vi "ICRA2024最后的ratio控制加轨迹跟踪.vi"() -> ()   [LabVIEW 2018]
doc: "Demonstrates the use of the Network Streams functions to send LED status to the myRIO target."
uses:
  <vilib>/Utility/file.llb/Read Delimited Spreadsheet (string).vi
  <vilib>/ErrorRing/Error Ring.xnode
  <vilib>/vision/NI_Vision_Development_Module.lvlib
panel:
  out "期望的ratio":dbl
  out "方向控制量":dbl
  out "速度控制量":dbl
  in  "分裂后的ratio":dbl
  in  "第二个desiredratio":dbl
  in  "第一个desiredratio":dbl
  in  "速度大小":dbl
  in  "终点纵坐标":dbl
  in  "终点横坐标":dbl
  out "实际纵坐标":sgl[](array[numeric])
  out "实际横坐标":sgl[](array[numeric])
  out "实际纵坐标":sgl
  out "实际横坐标":sgl
  out "方向d1":sgl
  out "轨迹跟踪点数":i32
  out "y":dbl
  out "x":dbl
  out "b":dbl[](array[numeric])
  in  "pp":dbl
  out "与目标点的距离":sgl
  in  "guiji":path=path "G:/ICRA-2024-Yuezhen Liu/Labview程序-ICRA2024-YuezhenLiu/small_myRIO_Helmholtz - 1111ke777/zgj轨迹delta为150.txt" caption="call7-8"
  out "Image 8":T1(plugin-control)
  out "ratio误差的绝对值":dbl[](array[numeric])
  in  "pd":dbl
  out "最终的ratio控制量":dbl
  in  "小p":dbl
  out "ratio误差的绝对值":dbl
  out "ratio的误差":dbl[](array[numeric])
  out "第二个前馈":dbl
  out "第一个前馈":dbl
  out "后一个ratio误差":dbl
  out "前一个ratio误差":dbl
  out "第一个i":i32
  out "ratio的误差":dbl
  out "裁剪后的二值图":T1(plugin-control)
  in  "布尔":bool
  in  "ribbon磁场开关":bool=TRUE
  out "面积":sgl[](array[numeric])
  out "面积":sgl
  out "数据总":dbl[][](array[numeric])
  out "i":i32[](array[numeric])
  out "aspect ratio":dbl[](array[numeric])
  out "D2":i32[](array[numeric])
  out "D1":i32[](array[numeric])
  out "field ratio":sgl[](array[numeric])
  out "field ratio":sgl=4.0
  out "时间":i32
  in  "打开数据记录":bool
  out "aspect ratio":dbl
  out "D2":i32
  out "D1":i32
  out "二值图":T1(plugin-control)
  in  "Search Rect (entire image)":T2={"Left"=200, "Top"=120, "Right"=2000, "Bottom"=1920, "Rotation"=0.0} {"Rotation" format="%.2f"; "Left" scale=0.0..1024.0; "Right" scale=0.0..1024.0}
  out "备用的椭圆角度":sgl
  in  "Number of Erosion":i32=10
  out "Image 7":T1(plugin-control)
  in  "Acquisition Control::Acquisition Frame Rate":dbl=19.50304412841797 min=1.4211589097976685 max=44.94382095336914
  out "Stopped":bool
  in  "Stop (F) 2":bool caption="Stop (F)"
  out "Objects 2":T3(array[cluster]) {"Aspect Ratio" format="%.2f"; "Orientation" format="%.2f"; "Area" format="%.2f"; "Object Center"."Y" format="%.2f"; "Object Center"."X" format="%.2f"}
  in  "Settings 2":T4={"Objects"=0, "Threshold"=128, "Reject Border"=FALSE, "Fill Holes"=FALSE, "Min Object Size"=FALSE, "Min Size"=20000, "Max Object Size"=FALSE, "Max Size"=100, "Show Search Area"=FALSE, "Show Center"=TRUE, "Show Bounding Box"=TRUE} {"Objects" items=["Bright Objects", "Dark Objects"]; "Threshold" min=1 max=999999999 step=1; "Max Size" min=1 max=999999999 step=1; "Min Size" min=1 max=999999999 step=1}
  in  "Range 2":cluster{"Lower value":sgl, "Upper value":sgl}={"Lower value"=0.0, "Upper value"=230.0} {"Upper value" format="%.2f"; "Lower value" format="%.2f"}
  in  "Pause":bool
  out "Array":dbl[](array[numeric])
  in  "Parameter Settings":T5(tab)=enum."Ribbon Oscillating Field" caption="Field Types"
  in  "fg":dbl
  in  "pg":dbl
  in  "dg":dbl
  in  "Ag":dbl
  in  "AoOF":dbl
  in  "fo":sgl
  in  "do":sgl
  in  "oo":sgl
  in  "po":sgl
  in  "cc":sgl
  in  "pc":sgl
  in  "wc":sgl
  in  "dc":sgl
  in  "Ac":dbl
  in  "pr":sgl
  in  "Ar":dbl=8.0
  in  "wr":sgl=18.0
  in  "dr":sgl
  in  "Dis phase step":dbl
  in  "Dis phase frequency (Hz)":dbl
  in  "Dis tumbling frequency (Hz)":dbl
  in  "Dis strength(mT)":dbl
  in  "Swa strength (mT)":dbl
  in  "Swa frequency (Hz)":dbl
  in  "Swa pitch angle (deg)":dbl
  in  "Swa direction angle (deg)":dbl
  in  "Swa ratio":dbl=1.0
  in  "Pitch Angle (rotating around Constant, deg)":dbl
  in  "Ratio (A/C)":sgl=4.0
  in  "Direction Angle (deg)":sgl
  in  "Pitch Angle (rotating around Origin, deg)":sgl
  in  "Frequency (Hz)":sgl=10.0
  in  "Strength (mT)":dbl=10.0
  in  "Ar 2":dbl=5.0 caption="Ar"
  in  "ratio":sgl=1.0
  in  "运动方向":sgl
  in  "长轴方向":sgl
  in  "wr  2":sgl=8.0
  in  "速度大小":sgl
  out "Numeric 5":i32
  in  "Stop":bool
  out "error out":errorcluster
  in  "Target IP Address":string="172.22.11.2"
  # "Overview: Magnetic field calculation, and send parameters to myRIO\nInstructions:\n1. Verify the value of Target IP Address. Set Visa resource name.\n2. Ensure RT Main.vi is already running. \n3. Run this VI. Set parameters of magnetic field."
  # "Strength (mT)"
  # "Pitch Angle (deg)"
  # "Direction Angle (deg)"
  # "Frequency (Hz)"
  # "Strength (mT)"
  # "Oscilation Frequency (Hz)"
  # "Oscilation Angle (deg)"
  # "Pitch Angle (deg)"
  # "Direction Angle (deg)"
  # "Strength (mT)"
  # "Frequency (Hz)"
  # "Pitch Angle (deg)"
  # "Direction Angle (deg)"
  # "Conical Angle (deg)"
  # "Strength (mT)"
  # "Frequency (Hz)"
  # "Pitch Angle (deg)"
  # "Direction Angle (deg)"
  # "Strength (mT)"
  # "Tumbling Frequency (Hz)"
  # "Phase Frequency (Hz)"
  # "Phase Step"
  # "Strength (mT)"
  # "Frequency (Hz)"
  # "Pitch Angle (deg)"
  # "Direction Angle (deg)"
  # "Ratio"
  # "Strength (mT)"
  # "Frequency (Hz)"
  # "Ratio (A/C)"
  # "Direction Angle (deg)"
  # "Pitch Angle (rotating around Origin, deg)"
  # "Pitch Angle (rotating around Constant, deg)"
  # "Strength (mT)"
  # "Frequency (Hz)"
  # "Pitch Angle  (deg)"
  # "longaxis"
  # "Direction Angle (deg)"
  # "ratio (l/s)"
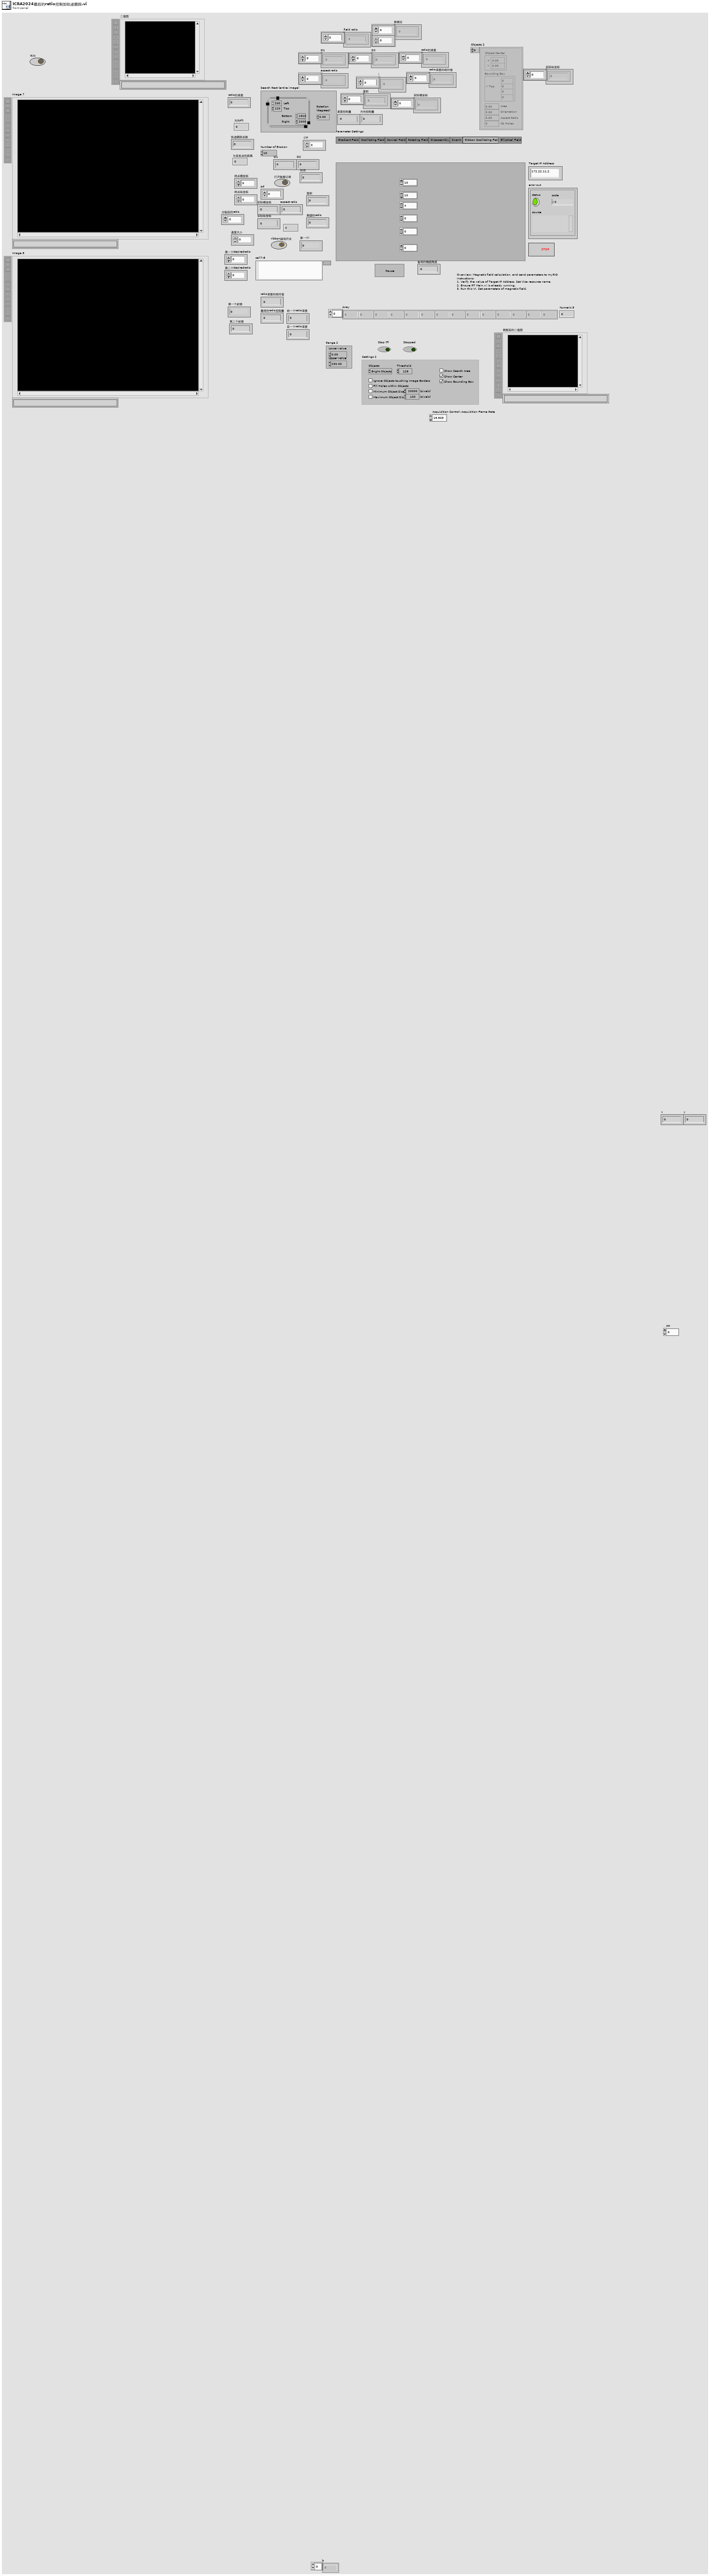
[diagram p1: front panel]
types:
  T1 = typedef "IMAQ Image.ctl" = refnum<image>
  T2 = typedef "IMAQ Rectangle" = cluster{"Left":i32, "Top":i32, "Right":i32, "Bottom":i32, "Rotation":dbl}
  T3 = cluster{"Object Center":cluster{"X":sgl, "Y":sgl}, "Bounding Box":cluster{"X Left":i32, "Y Top":i32, "X Right":i32, "Y Bottom":i32}, "Area":sgl, "Orientation":sgl, "Aspect Ratio":sgl, "Nb Holes":i32}[]
  T4 = cluster{"Objects":u16, "Threshold":i32, "Reject Border":bool, "Fill Holes":bool, "Min Object Size":bool, "Min Size":i32, "Max Object Size":bool, "Max Size":i32, "Show Search Area":bool, "Show Center":bool, "Show Bounding Box":bool}
  T5 = enum32{"Gradient Field ", "Oscillating Field", "Conical Field", "Rotating Field", "Disassembly", "Swarm", "Ribbon Oscillating Field", "Elliptical Field"}
  T6 = cluster{"Left":i32, "Top":i32, "Right":i32, "Bottom":i32}
  T7 = typedef "Image Type" = u32
  T8 = cluster{"Objects[0]":cluster{"Object Center":cluster{"X":sgl, "Y":sgl}, "Bounding Box":cluster{"X Left":i32, "Y Top":i32, "X Right":i32, "Y Bottom":i32}, "Area":sgl, "Orientation":sgl, "Aspect Ratio":sgl, "Nb Holes":i32}, "Objects[1]":cluster{"Object Center":cluster{"X":sgl, "Y":sgl}, "Bounding Box":cluster{"X Left":i32, "Y Top":i32, "X Right":i32, "Y Bottom":i32}, "Area":sgl, "Orientation":sgl, "Aspect Ratio":sgl, "Nb Holes":i32}, "Objects[2]":cluster{"Object Center":cluster{"X":sgl, "Y":sgl}, "Bounding Box":cluster{"X Left":i32, "Y Top":i32, "X Right":i32, "Y Bottom":i32}, "Area":sgl, "Orientation":sgl, "Aspect Ratio":sgl, "Nb Holes":i32}, "Objects[3]":cluster{"Object Center":cluster{"X":sgl, "Y":sgl}, "Bounding Box":cluster{"X Left":i32, "Y Top":i32, "X Right":i32, "Y Bottom":i32}, "Area":sgl, "Orientation":sgl, "Aspect Ratio":sgl, "Nb Holes":i32}, "Objects[4]":cluster{"Object Center":cluster{"X":sgl, "Y":sgl}, "Bounding Box":cluster{"X Left":i32, "Y Top":i32, "X Right":i32, "Y Bottom":i32}, "Area":sgl, "Orientation":sgl, "Aspect Ratio":sgl, "Nb Holes":i32}, "Objects[5]":cluster{"Object Center":cluster{"X":sgl, "Y":sgl}, "Bounding Box":cluster{"X Left":i32, "Y Top":i32, "X Right":i32, "Y Bottom":i32}, "Area":sgl, "Orientation":sgl, "Aspect Ratio":sgl, "Nb Holes":i32}, "Objects[6]":cluster{"Object Center":cluster{"X":sgl, "Y":sgl}, "Bounding Box":cluster{"X Left":i32, "Y Top":i32, "X Right":i32, "Y Bottom":i32}, "Area":sgl, "Orientation":sgl, "Aspect Ratio":sgl, "Nb Holes":i32}, "Objects[7]":cluster{"Object Center":cluster{"X":sgl, "Y":sgl}, "Bounding Box":cluster{"X Left":i32, "Y Top":i32, "X Right":i32, "Y Bottom":i32}, "Area":sgl, "Orientation":sgl, "Aspect Ratio":sgl, "Nb Holes":i32}, "Objects[8]":cluster{"Object Center":cluster{"X":sgl, "Y":sgl}, "Bounding Box":cluster{"X Left":i32, "Y Top":i32, "X Right":i32, "Y Bottom":i32}, "Area":sgl, "Orientation":sgl, "Aspect Ratio":sgl, "Nb Holes":i32}}
  T9 = cluster{"Object Center":cluster{"X":sgl, "Y":sgl}, "Bounding Box":cluster{"X Left":i32, "Y Top":i32, "X Right":i32, "Y Bottom":i32}, "Area":sgl, "Orientation":sgl, "Aspect Ratio":sgl, "Nb Holes":i32}
  T10 = cluster{"X Left":i32, "Y Top":i32, "X Right":i32, "Y Bottom":i32}
  T11 = typedef "ROI Descriptor" = cluster{"Global Rectangle":i32[], "Contours":cluster{"ID":enum32{"External", "Internal"}, "Type":u32, "Coordinates":i32[]}[]}
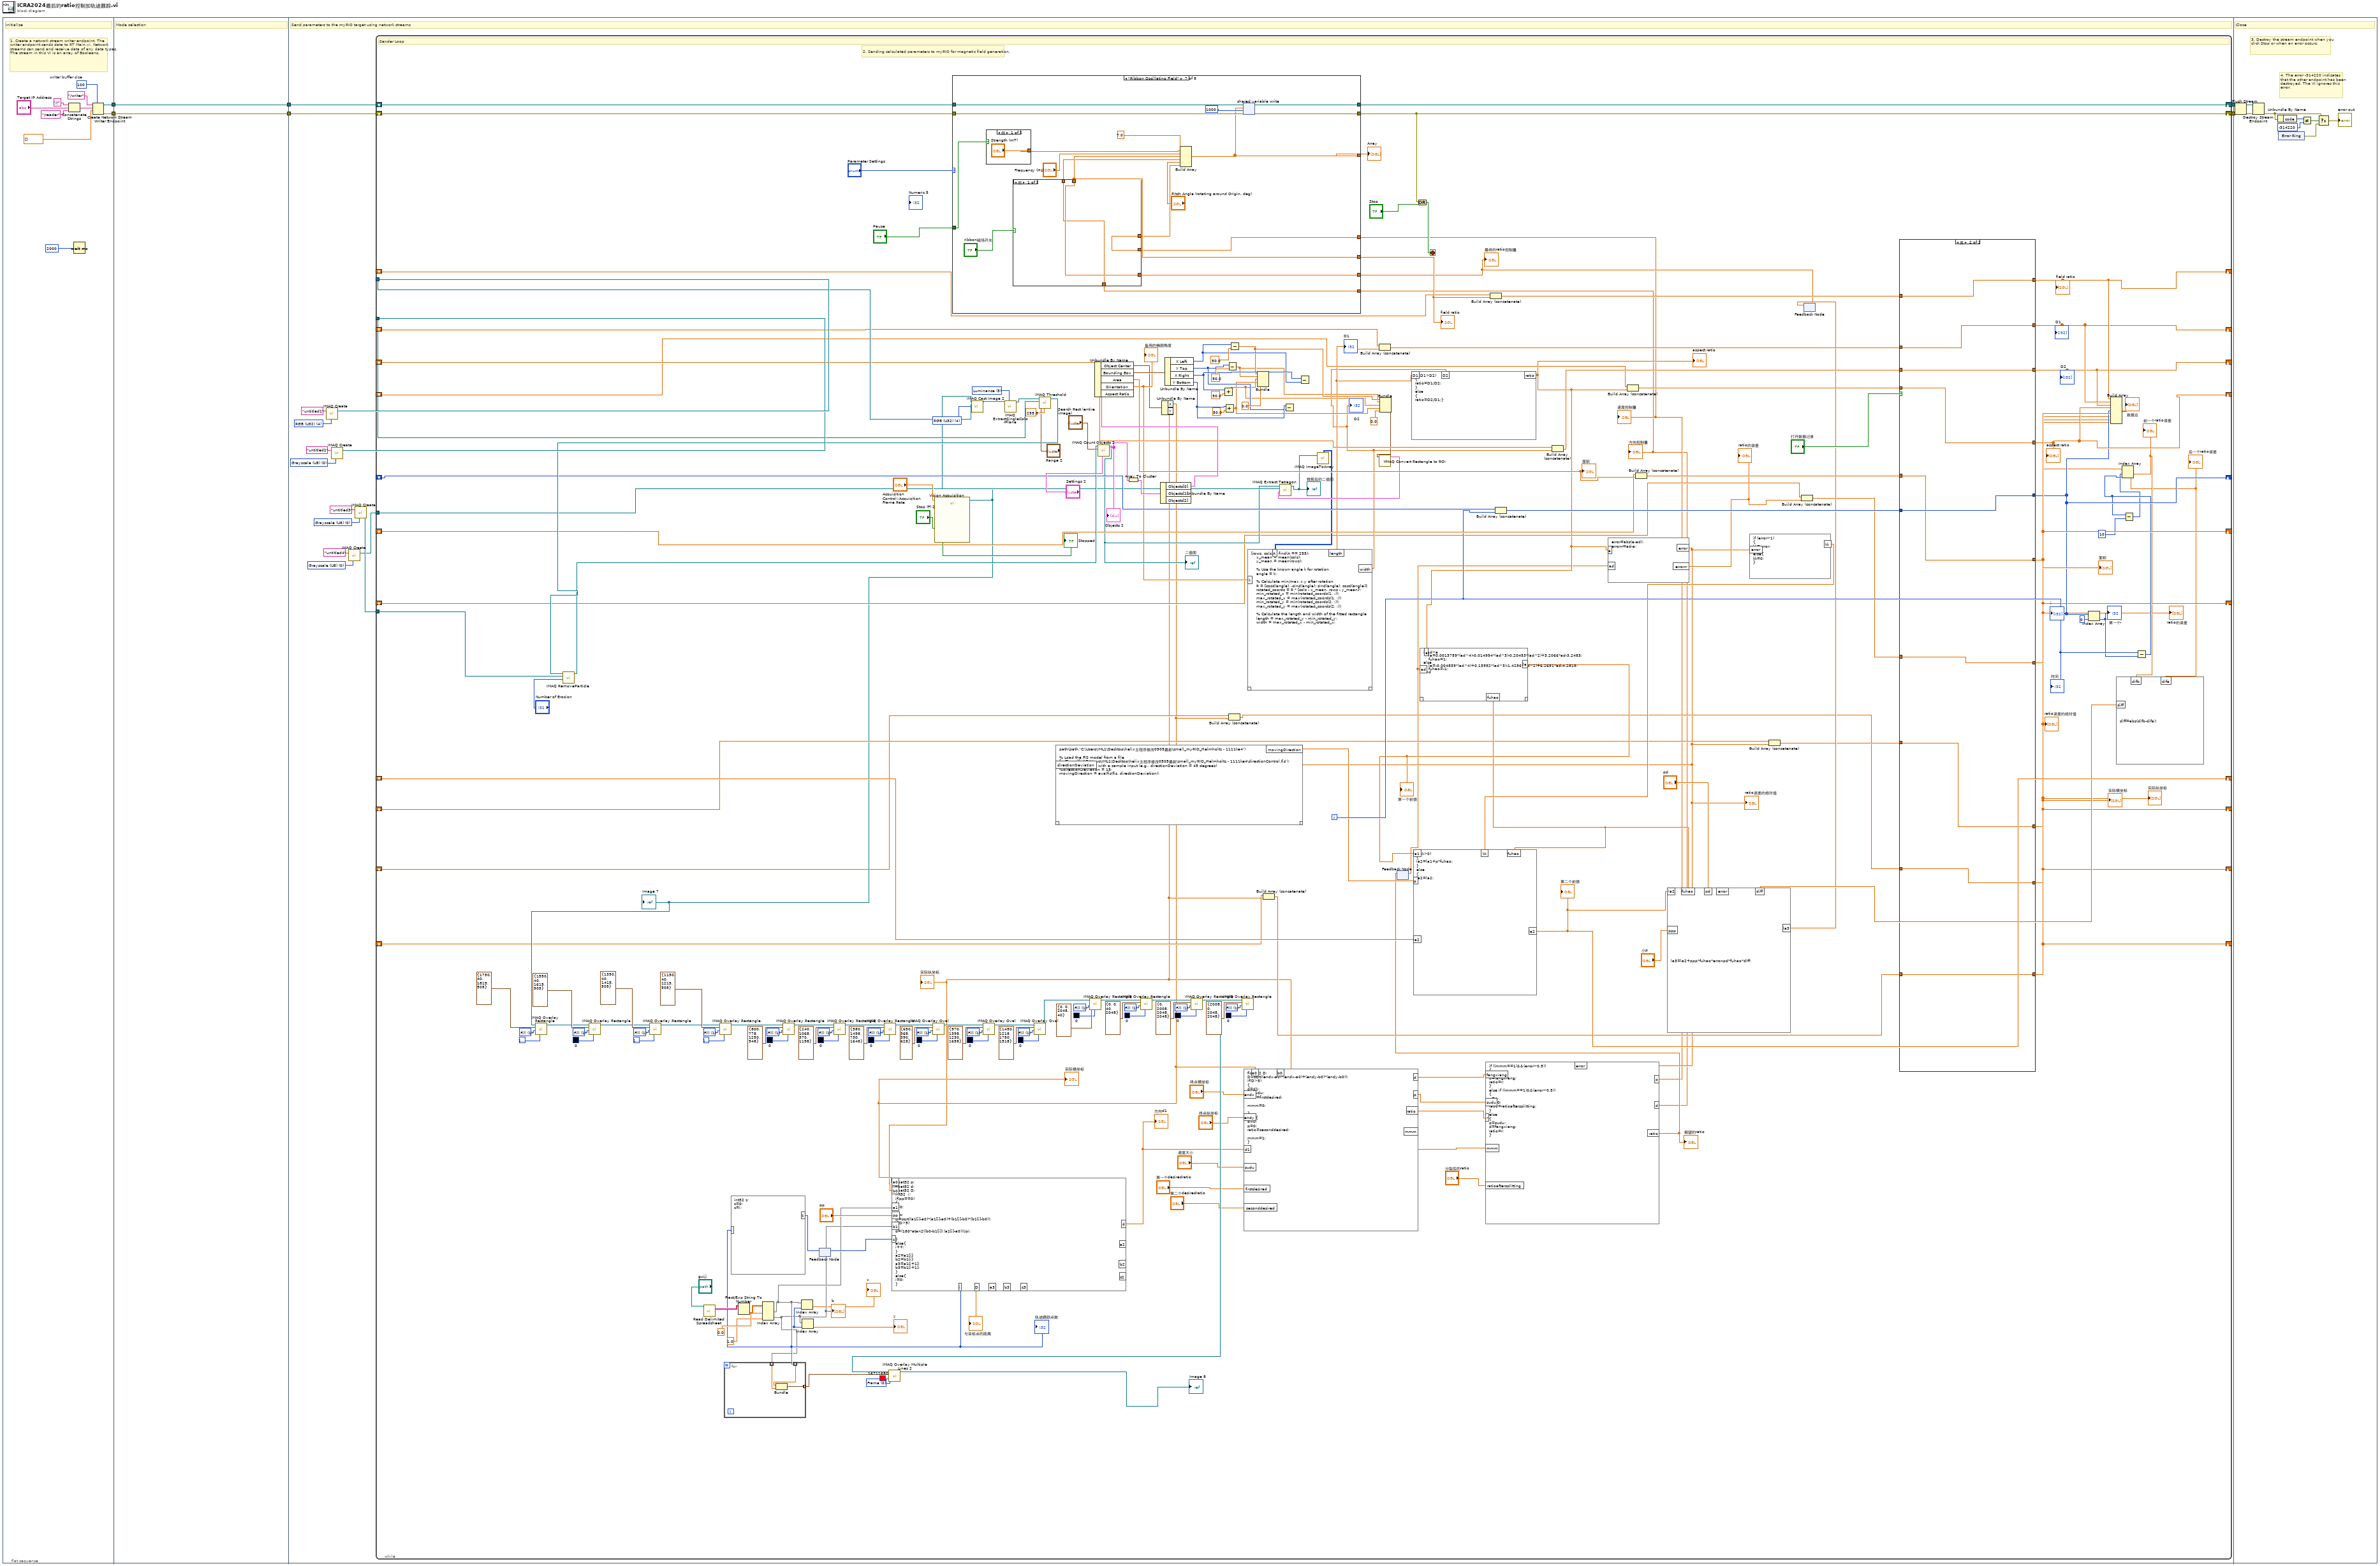
[diagram p0: block diagram]
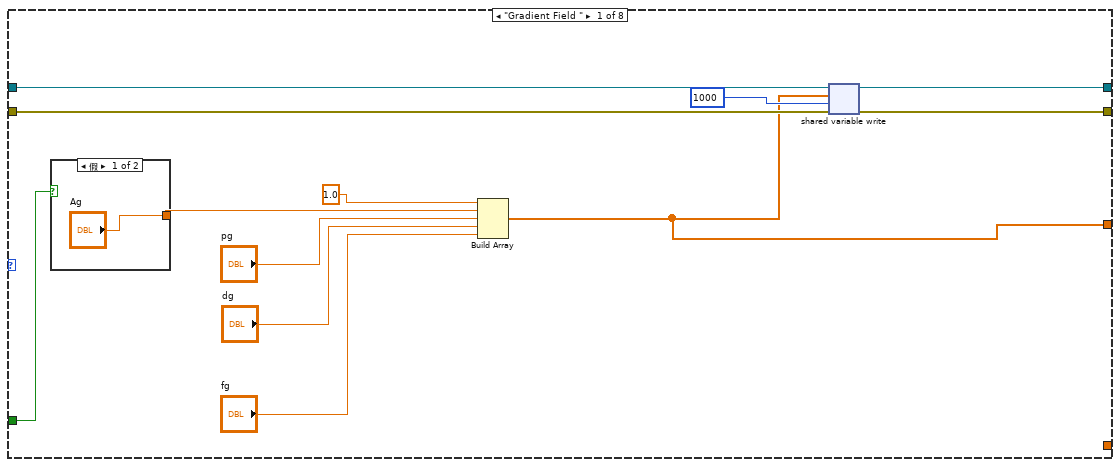
[diagram p3: hidden frame]
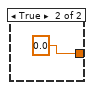
[diagram p4: hidden frame]
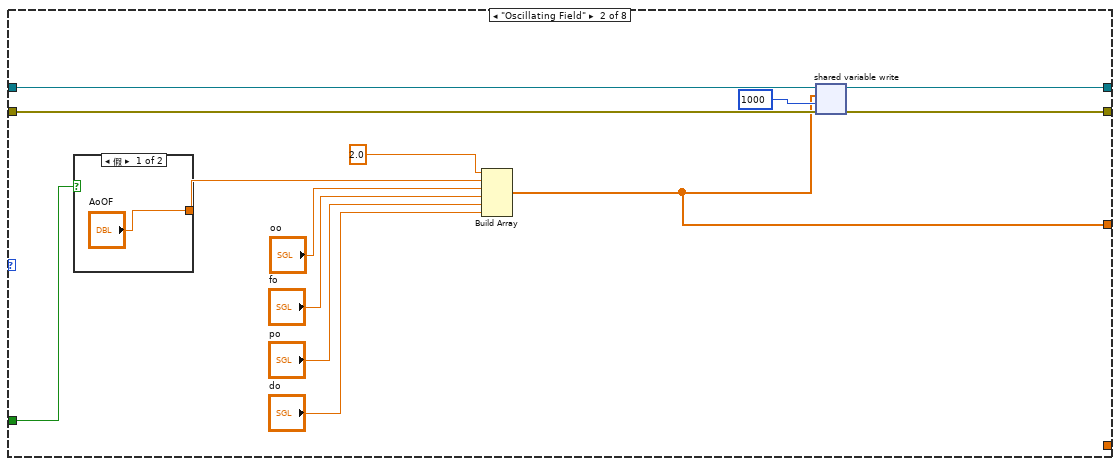
[diagram p5: hidden frame]
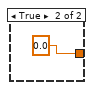
[diagram p6: hidden frame]
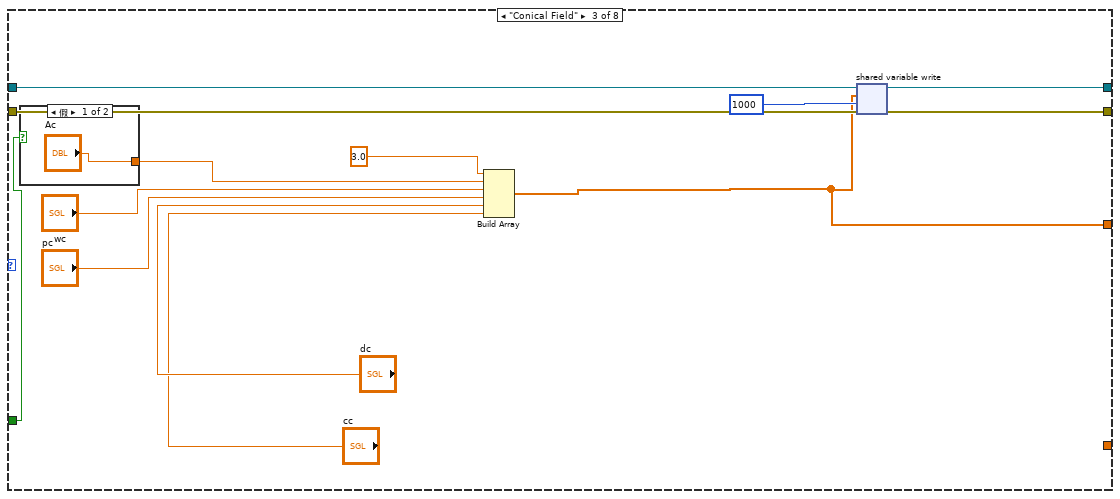
[diagram p7: hidden frame]
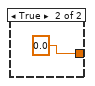
[diagram p8: hidden frame]
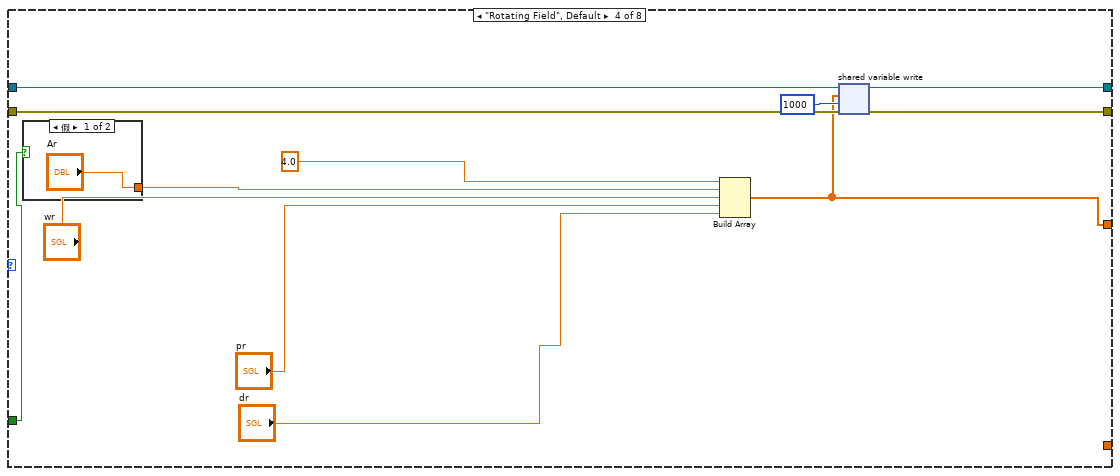
[diagram p9: hidden frame]
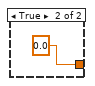
[diagram p10: hidden frame]
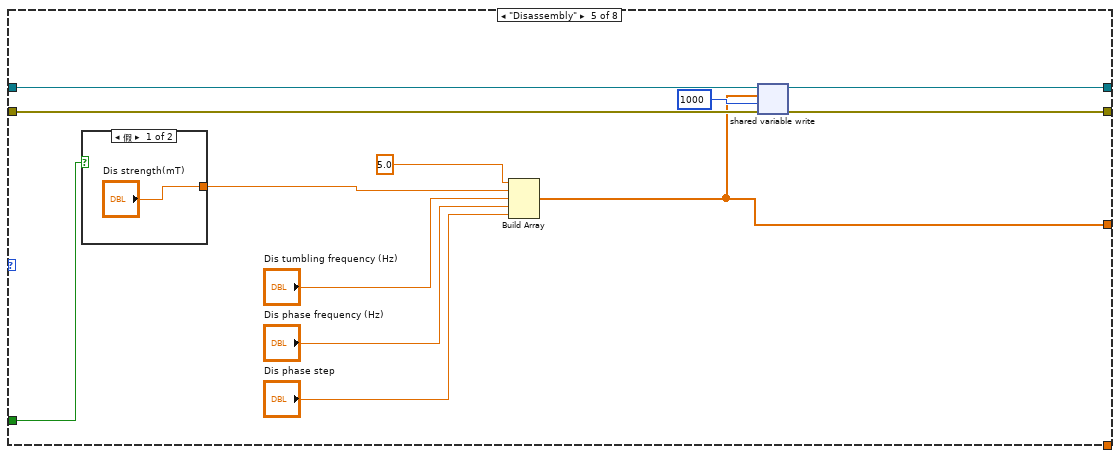
[diagram p11: hidden frame]
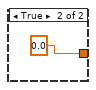
[diagram p12: hidden frame]
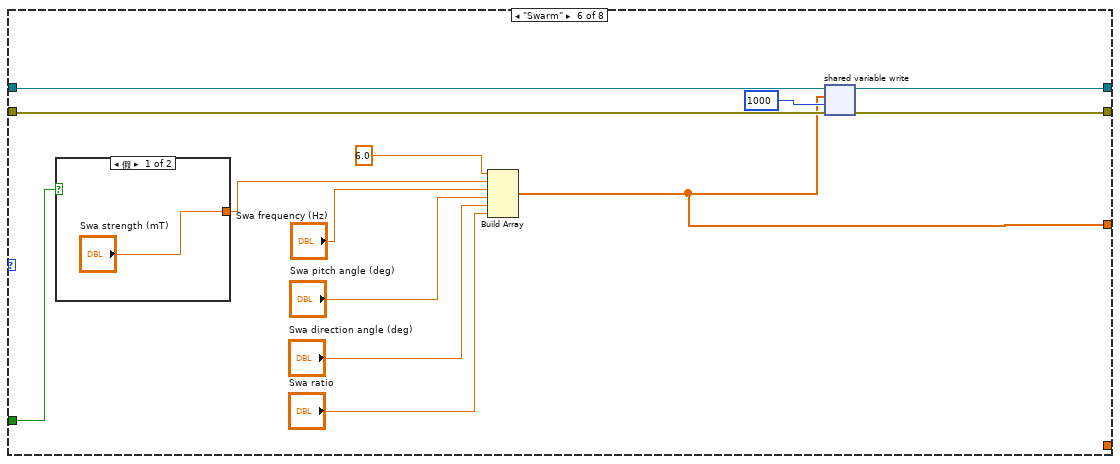
[diagram p13: hidden frame]
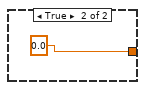
[diagram p14: hidden frame]
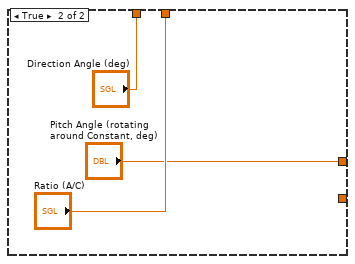
[diagram p15: hidden frame]
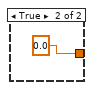
[diagram p16: hidden frame]
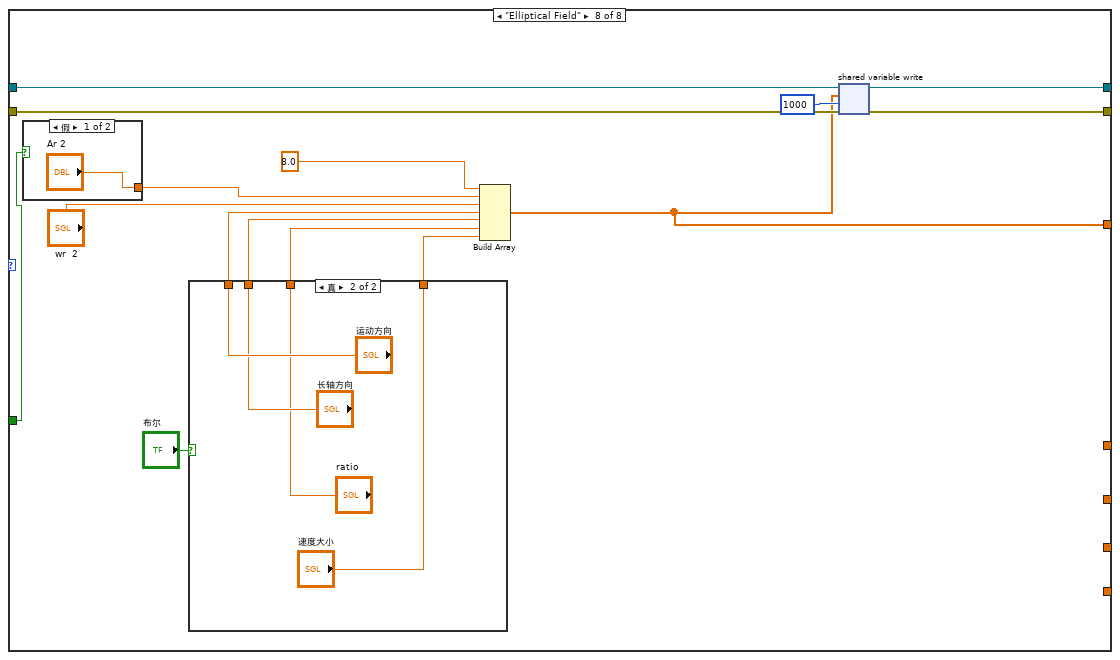
[diagram p17: hidden frame]
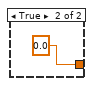
[diagram p19: hidden frame]
diagram:
  n1 = flat-sequence {
    tunnel: [w11] -> w2
    tunnel: [w10] -> w1
    tunnel: [w18] -> w4
    tunnel: [w17] -> w3
    tunnel: w1 -> [w17]
    tunnel: w2 -> [w18]
    tunnel: [w32] -> w6
    tunnel: w4 -> [w34]
    tunnel: [w31] -> w5
    tunnel: w3 -> [w33]
    tunnel: w6 -> [w393]
    tunnel: w5 -> [w390]
    frame #0 {
      w9 = 100  # writer buffer size
      # "1. Create a network stream writer endpoint. The writer endpoint sends data to RT Main.vi. Network streams can send and receive data of any data types. The stream in this VI is an array of Booleans."
      # "Initialize"
      n2 = Concatenate Strings("//", "Target IP Address", "/reader") -> (w16:string)
      n3 = Wait (ms)(milliseconds to wait=2000) -> ()  [unwired: 1 out]
      n4 = Create Network Stream Writer Endpoint(7:w9, 9:dbl[] [], 10:w16, 11:"/writer" ("reader name")) -> (0:w10:errorcluster, 3:w11:refnum<k21>)  [unwired: 3 in]
    }
    frame #1 {
      # "Mode selection"
    }
    frame #2 {
      w20 = T7 0 items=["Grayscale (U8)", "Grayscale (I16)", "Grayscale (SGL)", "Complex (CSG)", "RGB (U32)", "HSL (U32)", "RGB (U64)", "Grayscale (U16)"] ("Image Type")
      w23 = T7 0 items=["Grayscale (U8)", "Grayscale (I16)", "Grayscale (SGL)", "Complex (CSG)", "RGB (U32)", "HSL (U32)", "RGB (U64)", "Grayscale (U16)"] ("Image Type")
      w27 = T7 0 items=["Grayscale (U8)", "Grayscale (I16)", "Grayscale (SGL)", "Complex (CSG)", "RGB (U32)", "HSL (U32)", "RGB (U64)", "Grayscale (U16)"] ("Image Type")
      w29 = T7 4 items=["Grayscale (U8)", "Grayscale (I16)", "Grayscale (SGL)", "Complex (CSG)", "RGB (U32)", "HSL (U32)", "RGB (U64)", "Grayscale (U16)"] ("Image Type")
      # "Send parameters to the myRIO target using network streams"
      n5 = call "IMAQ Create"("Image Name"="untitled1", "Image Type"=w29) -> ("New Image"=w26:T1)  [unwired: 3 in, 1 out]
      n6 = call "IMAQ Create"("Image Name"="untitled2", "Image Type"=w27) -> ("New Image"=w25:T1)  [unwired: 3 in, 1 out]
      n7 = call "IMAQ Create"("Image Name"="untitled4", "Image Type"=w20) -> ("New Image"=w19:T1)  [unwired: 3 in, 1 out]
      n8 = call "IMAQ Create"("Image Name"="untitled3", "Image Type"=w23) -> ("New Image"=w22:T1)  [unwired: 3 in, 1 out]
      n9 = while {
        shift-right: [w232] -> w31
        shift-left: w33 -> [w234]
        shift-right: [w233] -> w32
        shift-left: w34 -> [w235]
        tunnel: w25 -> [w223]
        tunnel: w26 -> [w218]
        tunnel: w22 -> [w207]
        shift-right: [w185] -> _
        shift-left: _ -> [w194]
        shift-right: [w184] -> _
        shift-left: _ -> [w192]
        shift-right: [w183] -> _
        shift-left: _ -> [w190]
        shift-right: [w164] -> _
        shift-left: _ -> [w188]
        shift-right: [w163] -> _
        shift-left: _ -> [w186]
        shift-right: [w179] -> _
        shift-left: _ -> [w178]
        tunnel: w19 -> [w177]
        shift-right: [w153] -> _
        shift-left: _ -> [w154]
        shift-right: [w151] -> _
        shift-left: _ -> [w150]
        shift-right: [w135] -> _
        shift-left: _ -> [w136]
        shift-right: [w54] -> _
        shift-left: _ -> [w57]
        shift-right: [w53] -> _
        shift-left: _ -> [w55]
        i -> [w161]
        stop <- w222 stop-if-true
        w62 = u32 0 items=["Frame", "Fill"] ("Drawing Mode (Frame)")
        w81 = u32 1 items=["Frame", "Fill", "Highlight"] ("Drawing Mode (Frame)")
        w84 = u32 1 items=["Frame", "Fill", "Highlight"] ("Drawing Mode (Frame)")
        w87 = u32 1 items=["Frame", "Fill", "Highlight"] ("Drawing Mode (Frame)")
        w90 = u32 1 items=["Frame", "Fill", "Highlight"] ("Drawing Mode (Frame)")
        w97 = u32 1 items=["Frame", "Fill"] ("Drawing Mode (Frame)")
        w100 = u32 1 items=["Frame", "Fill"] ("Drawing Mode (Frame)")
        w105 = u32 1 items=["Frame", "Fill"] ("Drawing Mode (Frame)")
        w117 = u32 1 items=["Frame", "Fill", "Highlight"] ("Drawing Mode (Frame)")
        w110 = u32 1 items=["Frame", "Fill"] ("Drawing Mode (Frame)")
        w120 = u32 1 items=["Frame", "Fill", "Highlight"] ("Drawing Mode (Frame)")
        w125 = u32 1 items=["Frame", "Fill", "Highlight"] ("Drawing Mode (Frame)")
        w128 = u32 1 items=["Frame", "Fill", "Highlight"] ("Drawing Mode (Frame)")
        w131 = u32 1 items=["Frame", "Fill", "Highlight"] ("Drawing Mode (Frame)")
        w134 = u32 1 items=["Frame", "Fill", "Highlight"] ("Drawing Mode (Frame)")
        w217 = T7 4 items=["Grayscale (U8)", "Grayscale (I16)", "Grayscale (SGL)", "Complex (CSG)", "RGB (U32)", "HSL (U32)", "RGB (U64)", "Grayscale (U16)"] ("Image Type")
        w228 = 5 items=["Red", "Green", "Blue", "Hue", "Saturation", "Luminance", "Value", "Intensity"] ("Color Plane")
        # "2. Sending calculated parameters to myRIO for magnetic field generation."
        # "Sender Loop"
        n10 = call-poly <vilib>:"Read Delimited Spreadsheet.vi"("file path (dialog if empty)"="guiji") -> ("all rows"=w77:string[][])  [unwired: 9 in, 5 out]
        n11 = Fract/Exp String To Number(string=w77) -> (number=w76:dbl[][])  [unwired: 3 in, 1 out]
        n12 = Index Array(array=w76, index (col) #1=0.0, index (col) #2=1.0) -> (element #1=w69:dbl[], element #2=w67:dbl[])  [unwired: 2 in]
        "b" <- w67
        n13 = for {
          tunnel: w69 -> [w239] mode=indexing
          tunnel: w67 -> [w238] mode=indexing
          tunnel: [w237] -> w64 mode=indexing
          n14 = Bundle("String"=w239, "String"=w238) -> (w237:cluster{"String":dbl, "String":dbl})  [unwired: 1 in]
        }
        n15 = feedback #1() -> (w72:i32)  [unwired: 1 in]
        n16 = call "Vision Acquisition"("Acquisition Control::Acquisition Frame Rate"="Acquisition Control::Acquisition Frame Rate", "Stop (F)"="Stop (F) 2") -> ("Image Out"=w79:T1, "Stopped"=→"Stopped":bool)  [unwired: 23 in, 1 out]
        "Image 7" <- w79
        n17 = call "IMAQ Overlay Rectangle"("Color"=u32 16777222, "Drawing Mode (Frame)"=w128, "Rectangle"=T6 {"Left"=1750, "Top"=40, "Right"=1815, "Bottom"=505}, "Image"=w79) -> ("Image Out"=w108:T1)  [unwired: 6 in, 1 out]
        n18 = call "IMAQ Overlay Rectangle"("Color"=u32 0, "Drawing Mode (Frame)"=w125, "Rectangle"=T6 {"Left"=1550, "Top"=40, "Right"=1615, "Bottom"=505}, "Image"=w108) -> ("Image Out"=w122:T1)  [unwired: 6 in, 1 out]
        n19 = call "IMAQ Overlay Rectangle"("Color"=u32 16777222, "Drawing Mode (Frame)"=w131, "Rectangle"=T6 {"Left"=1350, "Top"=40, "Right"=1415, "Bottom"=505}, "Image"=w122) -> ("Image Out"=w121:T1)  [unwired: 6 in, 1 out]
        n20 = call "IMAQ Overlay Rectangle"("Color"=u32 16777222, "Drawing Mode (Frame)"=w134, "Rectangle"=T6 {"Left"=1150, "Top"=40, "Right"=1215, "Bottom"=505}, "Image"=w121) -> ("Image Out"=w109:T1)  [unwired: 6 in, 1 out]
        n21 = call "IMAQ Overlay Rectangle"("Color"=u32 0, "Drawing Mode (Frame)"=w120, "Rectangle"=T6 {"Left"=800, "Top"=778, "Right"=1250, "Bottom"=948}, "Image"=w109) -> ("Image Out"=w113:T1)  [unwired: 6 in, 1 out]
        n22 = call "IMAQ Overlay Rectangle"("Color"=u32 0, "Drawing Mode (Frame)"=w110, "Rectangle"=T6 {"Left"=240, "Top"=1068, "Right"=370, "Bottom"=1198}, "Image"=w113) -> ("Image Out"=w114:T1)  [unwired: 6 in, 1 out]
        n23 = call "IMAQ Overlay Rectangle"("Color"=u32 0, "Drawing Mode (Frame)"=w117, "Rectangle"=T6 {"Left"=580, "Top"=1498, "Right"=730, "Bottom"=1648}, "Image"=w114) -> ("Image Out"=w107:T1)  [unwired: 6 in, 1 out]
        n24 = call "IMAQ Overlay Oval"("Color"=u32 0, "Drawing Mode (Frame)"=w105, "Bounding Rectangle"=T6 {"Left"=650, "Top"=368, "Right"=390, "Bottom"=628}, "Image"=w107) -> ("Image Out"=w102:T1)  [unwired: 6 in, 1 out]
        n25 = call "IMAQ Cast Image 2"("Image Src"=w79, "Image Dst"=w218, "Image Type"=w217) -> ("Image Dst Out"=w219:T1)  [unwired: 11 in, 1 out]
        n26 = call "IMAQ Overlay Oval"("Color"=u32 0, "Drawing Mode (Frame)"=w100, "Bounding Rectangle"=T6 {"Left"=970, "Top"=1398, "Right"=1230, "Bottom"=1658}, "Image"=w102) -> ("Image Out"=w103:T1)  [unwired: 6 in, 1 out]
        n27 = call "IMAQ ExtractSingleColorPlane"("Color Plane"=w228, "Image Src"=w219) -> ("Image Dst Out"=w205:T1)  [unwired: 8 in, 1 out]
        n28 = call "IMAQ Overlay Oval"("Color"=u32 0, "Drawing Mode (Frame)"=w97, "Bounding Rectangle"=T6 {"Left"=1450, "Top"=1218, "Right"=1750, "Bottom"=1518}, "Image"=w103) -> ("Image Out"=w95:T1)  [unwired: 6 in, 1 out]
        n29 = call "IMAQ Threshold"("Replace Value"=sgl 255.0, "Range"="Range 2", "Image Dst"=w223, "Image Src"=w205) -> ("Image Dst Out"=w208:T1)  [unwired: 6 in, 1 out]
        n30 = call "IMAQ RemoveParticle"("Number of Erosion"="Number of Erosion", "Image Dst"=w207, "Image Src"=w208) -> ("Image Dst Out"=w200:T1)  [unwired: 7 in, 1 out]
        n31 = call "IMAQ Overlay Rectangle"("Color"=u32 0, "Drawing Mode (Frame)"=w90, "Rectangle"=T6 {"Left"=0, "Top"=0, "Right"=2048, "Bottom"=40}, "Image"=w95) -> ("Image Out"=w94:T1)  [unwired: 6 in, 1 out]
        n32 = call "IMAQ Count Objects 2"("Settings"="Settings 2", "Search Rect (entire image)"="Search Rect (entire image)", "Image"=w200) -> ("Image Out"=w176:T1, "Objects"=w224:T3)  [unwired: 4 in, 3 out]
        "Objects 2" <- w224
        "二值图" <- w176
        n33 = Array To Cluster(array=w224) -> (cluster=w210:T8)
        n34 = call "IMAQ Overlay Rectangle"("Color"=u32 0, "Drawing Mode (Frame)"=w87, "Rectangle"=T6 {"Left"=0, "Top"=0, "Right"=40, "Bottom"=2048}, "Image"=w94) -> ("Image Out"=w93:T1)  [unwired: 6 in, 1 out]
        n35 = Unbundle By Name(w210) -> ("Objects[0]"=w209:T9)  [unwired: 2 out]
        n36 = Unbundle By Name(w209) -> ("Object Center"=w59:cluster{"X":sgl, "Y":sgl}, "Bounding Box"=w216:T10, "Area"=w181:sgl, "Orientation"=w159:sgl)  [unwired: 1 out]
        "备用的椭圆角度" <- w159
        "面积" <- w181
        n37 = Unbundle By Name(w59) -> ("X"=w48:sgl, "Y"=w47:sgl)
        "实际横坐标" <- w48
        "实际纵坐标" <- w47
        n38 = formula code="float32 p;\nfloat32 d;\nfloat32 D;\nint32  i;\nif(pp==0)\n{\ni=0;\n\ni=z;\nD=sqrt((a1[i]-a0)*(a1[i]-a0)+(b1[i]-b0)*(b1[i]-b0));\nif(D>5)\n{\nd=(180*atan2((b0-b1[i]),(a1[i]-a0)))/pi;\n\n}\nelse{\ni++;\n}\na2=a1[i];\nb2=b1[i];\na3=a1[i+1];\nb3=b1[i+1];\n}\nelse{\ni=0;\n}"("a0"=w48, "b0"=w47, "a1"=w69, "b1"=w67, "z"=w72, "pp"="pp") -> ("i"=w68:i32, "D"=→"与目标点的距离":sgl, "d"=w50:sgl)  [unwired: 6 out]
        "轨迹跟踪点数" <- w68
        "方向d1" <- w50
        n39 = formula code="int32 z;\nz=0;\nz=i;"("i"=w68) -> ("z"=w73:i32)
        n40 = Index Array(array=w69, index=w68) -> (element=→"x":dbl)
        n41 = Index Array(array=w67, index=w68) -> (element=→"y":dbl)
        n42 = feedback-in #1(w73) -> ()
        n43 = Unbundle By Name(w216) -> ("X Left"=w202:i32, "Y Top"=w198:i32, "X Right"=w203:i32, "Y Bottom"=w199:i32)
        n44 = call "IMAQ Overlay Rectangle"("Color"=u32 0, "Drawing Mode (Frame)"=w84, "Rectangle"=T6 {"Left"=0, "Top"=2008, "Right"=2048, "Bottom"=2048}, "Image"=w93) -> ("Image Out"=w92:T1)  [unwired: 6 in, 1 out]
        n45 = Add(x=w203, y=50.0) -> (x+y=w171:dbl)
        n46 = Add(x=w199, y=50.0) -> (x+y=w170:dbl)
        n47 = Subtract(x=w198, y=50.0) -> (x-y=w172:dbl)
        n48 = Build Array (concatenate)(w57, w48) -> (w58:sgl[])
        n49 = Subtract(x=w202, y=50.0) -> (x-y=w173:dbl)
        n50 = call "IMAQ Overlay Rectangle"("Color"=u32 0, "Drawing Mode (Frame)"=w81, "Rectangle"=T6 {"Left"=2008, "Top"=0, "Right"=2048, "Bottom"=2048}, "Image"=w92) -> ("Image Out"=w61:T1)  [unwired: 6 in, 1 out]
        n51 = call "IMAQ Overlay Multiple Lines 2"("Image"=w61, "Line End Points"=w64, "Drawing Mode (Frame)"=w62, "Color"=u32 16711680) -> ("Image Out"=→"Image 8":T1)  [unwired: 10 in, 1 out]
        n52 = formula code="float32 D;\nD=sqrt((endx-a0)*(endx-a0)+(endy-b0)*(endy-b0));\nif(D>5)\n{\nd=d1;\np=sudu;\nratio=firstdesired;\n\nmmm=0;\n\n}\nelse{\nd=0;\np=0;\nratio=seconddesired;\n\nmmm=1;\n}"("endx"="终点横坐标", "endy"="终点纵坐标", "d1"=w50, "sudu"="速度大小", "firstdesired"="第一个desiredratio", "seconddesired"="第二个desiredratio", "a0"=w48, "b0"=w47) -> ("p"=w43:dbl, "ratio"=w41:dbl, "d"=w42:dbl, "mmm"=w44:dbl)
        n53 = Bundle(w173, w172, w171, w170, 0.0) -> ()  [unwired: 1 in, 1 out]
        n54 = Build Array (concatenate)(w55, w47) -> (w56:sgl[])
        n55 = Subtract(x=w199, y=w198) -> ()  [unwired: 1 out]
        n56 = Subtract(x=w203, y=w202) -> ()  [unwired: 1 out]
        n57 = Bundle(w173, w172, w171, w170, 0.0) -> (w168:cluster{dbl, dbl, dbl, dbl, dbl})  [unwired: 1 in]
        n58 = call "IMAQ Convert Rectangle to ROI"("Rectangle"=w168) -> ("ROI Descriptor"=w174:T11)  [unwired: 8 in, 1 out]
        n59 = call-poly "IMAQ Extract Tetragon"("ROI Descriptor"=w174, "Image Dst"=w177, "Image Src"=w176) -> ("Image Dst Out"=w175:T1)  [unwired: 7 in, 1 out]
        "裁剪后的二值图" <- w175
        n60 = call "IMAQ ImageToArray"("Image"=w175) -> ("Image Pixels (U8)"=w167:u8[][])  [unwired: 3 in, 4 out]
        n61 = script code="[rows, cols] = find(A == 255);\n    x_mean = mean(cols);\n    y_mean = mean(rows);\n\n    % Use the known angle k for rotation\n    angle = k;\n\n    % Calculate min/max x,y after rotation\n    R = [cosd(angle), -sind(angle); sind(angle), cosd(angle)];\n    rotated_coords = R * [cols - x_mean, rows - y_mean]';\n    min_rotated_x = min(rotated_coords(1, :));\n    max_rotated_x = max(rotated_coords(1, :));\n    min_rotated_y = min(rotated_coords(2, :));\n    max_rotated_y = max(rotated_coords(2, :));\n\n    % Calculate the length and width of the fitted rectangle\n    length = max_rotated_y - min_rotated_y;\n    width = max_rotated_x - min_rotated_x;"("A"=w167, "k"=w159) -> ("length"=w166:dbl, "width"=w165:dbl)  [unwired: 1 in, 1 out]
        "D1" <- w166
        "D2" <- w165
        n62 = Build Array (concatenate)(w192, w166) -> (w193:dbl[])
        n63 = feedback #2() -> (w37:dbl)  [unwired: 1 in]
        n64 = formula code="if (D1>D2)\n{\nratio=D1/D2;\n}\nelse\n{\nratio=D2/D1;}"("D1"=w166, "D2"=w165) -> ("ratio"=w139:dbl)
        "aspect ratio" <- w139
        n65 = script code="if ad>a\n    la=0.0013759*(ad^4)-0.014994*(ad^3)-0.20453*(ad^2)+3.2066*ad-3.2483;\n    fuhao=1;\nelse\n    la=-0.004839*(ad^4)+0.13992*(ad^3)-1.4256*(ad^2)+6.2651*ad-4.2815;\n    fuhao=-1;\nend"("a"=w139, "ad"=w37) -> ("la"=w141:dbl, "fuhao"=w140:dbl)  [unwired: 1 in, 1 out]
        "第一个前馈" <- w141
        n66 = Build Array (concatenate)(w186, w161) -> (w187:i32[])
        n67 = Build Array (concatenate)(w190, w165) -> (w191:dbl[])
        n68 = formula code="error=abs(a-ad);\nerrorrr=ad-a;"("a"=w139, "ad"=w37) -> ("error"=w40:dbl, "errorrr"=w146:dbl)
        "ratio的误差" <- w146
        "ratio误差的绝对值" <- w40
        n69 = script code="path(path,'C:\\Users\\IML1\\Desktop\\helix主程序修改0505最新\\small_myRIO_Helmholtz - 1111ke4')\n\n% Load the FIS model from a file\nfis = readfis('C:\\Users\\IML1\\Desktop\\helix主程序修改0505最新\\small_myRIO_Helmholtz - 1111ke4\\directionControl.fis');\n% Evaluate the FIS with a sample input (e.g., directionDeviation = 45 degrees)\n%directionDeviation = 15;\nmovingDirection = evalfis(fis, directionDeviation);"("directionDeviation"=w40) -> ("movingDirection"=w138:dbl)  [unwired: 1 in, 1 out]
        n70 = formula code="if ((mmm==1)&&(error>0.5))\n{\np=sudu;\nd=fangxiang;\nratio=r;\n}\nelse if ((mmm==1)&&(error<0.5))\n{\np=4;\nd=90;\nratio=ratioaftersplitting;\n}\nelse\n{\np=sudu;\nd=fangxiang;\nratio=r;\n}"("mmm"=w44, "sudu"=w43, "fangxiang"=w42, "r"=w41, "error"=w40, "ratioaftersplitting"="分裂后的ratio") -> ("p"=w36:dbl, "d"=w35:dbl, "ratio"=w38:dbl)
        "速度控制量" <- w36
        "方向控制量" <- w35
        "期望的ratio" <- w38
        n71 = feedback-in #2(w38) -> ()
        n72 = Build Array (concatenate)(w188, w139) -> (w189:dbl[])
        n73 = Build Array (concatenate)(w178, w181) -> (w180:sgl[])
        n74 = formula code="if (error>1)\n{\nkk=error;\n}\nelse{\nkk=0;\n}"("error"=w40) -> ("kk"=w155:dbl)
        n75 = formula code="if(kk>0)\n{\nla2=la1+p*fuhao;\n}\nelse\n{\nla2=la2;\n}"("kk"=w155, "la1"=w141, "fuhao"=w140, "p"=w138, "la2"=w154) -> ("la2"=w153:dbl)
        "第二个前馈" <- w153
        n76 = Build Array (concatenate)(w136, w40) -> (w137:dbl[])
        n77 = Build Array (concatenate)(w150, w146) -> (w152:dbl[])
        n78 = feedback #3() -> (w143:dbl)  [unwired: 1 in]
        "最终的ratio控制量" <- w143
        n79 = case shown="\"Ribbon Oscillating Field\"" "Parameter Settings" {
          tunnel: w235 -> [w260 w275 w290 w304 w318 w332 w354 w376]
          tunnel: w234 -> [w257 w274 w289 w303 w316 w331 w352 w375]
          tunnel: [w259 w273 w287 w302 w317 w330 w353 w374] -> w233
          tunnel: [w258 w272 w288 w301 w315 w329 w351 w373] -> w232
          tunnel: [w253 w266 w281 w296 w309 w324 w349 w368] -> w231
          tunnel: "Pause" -> [w251 w264 w279 w294 w308 w323 w346 w366]
          tunnel: [_ _ _ _ _ _ w344 _] -> w196
          tunnel: w143 -> [_ _ _ _ _ _ w341 _]
          tunnel: w36 -> [_ _ _ _ _ _ w338 _]
          tunnel: w35 -> [_ _ _ _ _ _ w337 _]
          frame "Gradient Field " {
            n80 = case shown="假" w251 {
              tunnel: ["Ag" 0.0] -> w252
              frame False {
              }
              frame True {
              }
            }
            n81 = Build Array(1.0, w252, "pg", "dg", "fg") -> (w253:dbl[])
            n82 = shared-variable-write(w260, w257, w253, 1000 ("timeout ms (-1)")) -> (w259:refnum<k21>, w258:errorcluster)  [unwired: 1 out]
          }
          frame "Oscillating Field" {
            n83 = case shown="假" w264 {
              tunnel: ["AoOF" 0.0] -> w265
              frame False {
              }
              frame True {
              }
            }
            n84 = Build Array(2.0, w265, "oo", "fo", "po", "do") -> (w266:dbl[])
            n85 = shared-variable-write(w275, w274, w266, 1000 ("timeout ms (-1)")) -> (w273:refnum<k21>, w272:errorcluster)  [unwired: 1 out]
          }
          frame "Conical Field" {
            # "FG"
            n86 = case shown="假" w279 {
              tunnel: ["Ac" 0.0] -> w280
              frame False {
              }
              frame True {
              }
            }
            n87 = Build Array(3.0, w280, "wc", "pc", "dc", "cc") -> (w281:dbl[])
            n88 = shared-variable-write(w290, w289, w281, 1000 ("timeout ms (-1)")) -> (w287:refnum<k21>, w288:errorcluster)  [unwired: 1 out]
          }
          frame "Rotating Field", Default {
            n89 = case shown="假" w294 {
              tunnel: ["Ar" 0.0] -> w295
              frame False {
              }
              frame True {
              }
            }
            n90 = Build Array(4.0, w295, "wr", "pr", "dr") -> (w296:dbl[])
            n91 = shared-variable-write(w304, w303, w296, 1000 ("timeout ms (-1)")) -> (w302:refnum<k21>, w301:errorcluster)  [unwired: 1 out]
          }
          frame "Disassembly" {
            n92 = case shown="假" w308 {
              tunnel: ["Dis strength(mT)" 0.0] -> w313
              frame False {
              }
              frame True {
              }
            }
            n93 = Build Array(5.0, w313, "Dis tumbling frequency (Hz)", "Dis phase frequency (Hz)", "Dis phase step") -> (w309:dbl[])
            n94 = shared-variable-write(w318, w316, w309, 1000 ("timeout ms (-1)")) -> (w317:refnum<k21>, w315:errorcluster)  [unwired: 1 out]
          }
          frame "Swarm" {
            n95 = case shown="假" w323 {
              tunnel: ["Swa strength (mT)" 0.0] -> w322
              frame False {
              }
              frame True {
              }
            }
            n96 = Build Array(6.0, w322, "Swa frequency (Hz)", "Swa pitch angle (deg)", "Swa direction angle (deg)", "Swa ratio") -> (w324:dbl[])
            n97 = shared-variable-write(w332, w331, w324, 1000 ("timeout ms (-1)")) -> (w330:refnum<k21>, w329:errorcluster)  [unwired: 1 out]
          }
          frame "Ribbon Oscillating Field" {
            n98 = case shown="假" w346 {
              tunnel: ["Strength (mT)" 0.0] -> w345
              frame False {
              }
              frame True {
              }
            }
            n99 = case shown="假" "ribbon磁场开关" {
              tunnel: [w357 "Ratio (A/C)"] -> w344
              tunnel: w341 -> [w357 _]
              tunnel: [w355 "Direction Angle (deg)"] -> w340
              tunnel: [w356 "Pitch Angle (rotating around Constant, deg)"] -> w339
              tunnel: w338 -> [w356 _]
              tunnel: w337 -> [w355 _]
              frame False {
              }
              frame True {
              }
            }
            n100 = Build Array(7.0, w345, "Frequency (Hz)", w344, w340, "Pitch Angle (rotating around Origin, deg)", w339) -> (w349:dbl[])
            n101 = shared-variable-write(w354, w352, w349, 1000 ("timeout ms (-1)")) -> (w353:refnum<k21>, w351:errorcluster)  [unwired: 1 out]
          }
          frame "Elliptical Field" {
            n102 = case shown="假" w366 {
              tunnel: ["Ar 2" 0.0] -> w367
              frame False {
              }
              frame True {
              }
            }
            n103 = case shown="真" "布尔" {
              tunnel: [_ "运动方向"] -> w371
              tunnel: [_ "长轴方向"] -> w370
              tunnel: [_ "ratio"] -> w365
              tunnel: [_ "速度大小"] -> w364
              frame False {
              }
              frame True {
              }
            }
            n104 = Build Array(8.0, w367, "wr  2", w371, w370, w365, w364) -> (w368:dbl[])
            n105 = shared-variable-write(w376, w375, w368, 1000 ("timeout ms (-1)")) -> (w374:refnum<k21>, w373:errorcluster)  [unwired: 1 out]
          }
        }
        "Array" <- w231
        "field ratio" <- w196
        n106 = Or(x=w232, y="Stop") -> (x .or. y?=w222:bool)
        n107 = Build Array (concatenate)(w194, w196) -> (w195:dbl[])
        n108 = case shown="真" "打开数据记录" {
          tunnel: [_ w249] -> w185
          tunnel: w195 -> [_ w249]
          tunnel: [_ w248] -> w184
          tunnel: w193 -> [_ w248]
          tunnel: [_ w247] -> w183
          tunnel: w191 -> [_ w247]
          tunnel: [_ w246] -> w164
          tunnel: w189 -> [_ w246]
          tunnel: [_ w245] -> w163
          tunnel: w187 -> [_ w245]
          tunnel: [_ w244] -> w179
          tunnel: w180 -> [_ w244]
          tunnel: [_ w243] -> w151
          tunnel: w152 -> [_ w243]
          tunnel: [_ w242] -> w135
          tunnel: w137 -> [_ w242]
          tunnel: [_ w241] -> w54
          tunnel: w58 -> [_ w241]
          tunnel: [_ w240] -> w53
          tunnel: w56 -> [_ w240]
          frame False {
          }
          frame True {
          }
        }
        "field ratio" <- w185
        "D1" <- w184
        "D2" <- w183
        "aspect ratio" <- w164
        "i" <- w163
        "面积" <- w179
        "ratio的误差" <- w151
        "ratio误差的绝对值" <- w135
        "实际横坐标" <- w54
        "实际纵坐标" <- w53
        n109 = Index Array(array=w163, index=0 ("索引")) -> (element=w160:i32)
        "第一个i" <- w160
        n110 = Build Array(w185, w184, w183, w164, w163, w179, w135, w54, w53) -> (→"数据总":dbl[][])
        n111 = Subtract(x=w161, y=w160) -> (x-y=w158:i32)
        n112 = Subtract(x=w158, y=10) -> (x-y=w157:i32)
        n113 = Index Array(array=w151, index #1=w157, index #2=w158) -> (element #1=w149:dbl, element #2=w148:dbl)
        "前一个ratio误差" <- w149
        "后一个ratio误差" <- w148
        n114 = formula code="diff=abs(difb-difa);"("difb"=w149, "difa"=w148) -> ("diff"=w147:dbl)
        n115 = formula code="la3=la2+ppp*fuhao*error-pd*fuhao*diff;"("la2"=w153, "fuhao"=w140, "diff"=w147, "ppp"="小p", "pd"="pd", "error"=w40) -> ("la3"=w144:dbl)
        n116 = feedback-in #3(w144) -> ()
        "时间" <- w161
      }
    }
    frame #3 {
      # "4. The error -314220 indicates that the other endpoint has been destroyed. The VI ignores this error."
      # "3. Destroy the stream endpoint when you click Stop or when an error occurs."
      # "Close"
      n117 = Flush Stream(8:w390, 11:w393) -> (0:w391:errorcluster, 3:w392:refnum<k21>)  [unwired: 2 in, 1 out]
      n118 = Destroy Stream Endpoint(8:w391, 11:w392) -> (0:w385:errorcluster)
      n119 = Unbundle By Name(w385) -> ("code"=w389:i32)
      n120 = xnode "Error Ring"() -> ("错误输出"=w386:errorcluster)
      n121 = Not Equal?(x=w389, y=-314220) -> (x != y?=w387:bool)
      n122 = Select(t=w385, s=w387, f=w386) -> (s? t:f=→"error out":errorcluster)
    }
  }
